vi "Teleop.vi"(10 "Match Info":T1={"Autonomous Elapsed Seconds"=0.0, "TeleOp Elapsed Seconds"=0.0, "Disabled Elapsed Seconds"=0.0, "Visited Autonomous"=FALSE, "Visited TeleOp"=FALSE, "Visited Disabled"=FALSE, "Autonomous Settings"={"Autonomous Style"=enum."Independent", "VI Refnum"=refnum}}, 11 "Call Context":T2) -> ()   [LabVIEW 2018]
doc: "This VI is called for each enabled TeleOp packet received from the DS. It is typically used to read from joysticks and other inputs and update I/O or setpoints for timed control loops. It should complete and return within 20 milliseconds or risk missing DS packets."
uses:
  <vilib>/Rock Robotics/WPI/DriverStation/WPI_DriverStationDerivedRobotMode.ctl
  <vilib>/Rock Robotics/WPI/DriverStation/WPI_DriverStationMatch Info.ctl
  <vilib>/Rock Robotics/WPI/Joystick/WPI_JoystickDeviceEnum.ctl
  <vilib>/addons/control/pid/pid.llb/PID (DBL).vi
  <vilib>/addons/control/pid/NI_PID_pid.lvlib
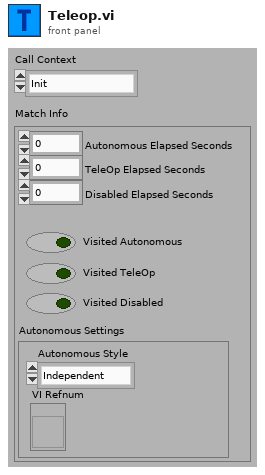
[diagram p1: front panel]
types:
  T1 = typedef "WPI_DriverStationMatch Info.ctl" = cluster{"Autonomous Elapsed Seconds":dbl, "TeleOp Elapsed Seconds":dbl, "Disabled Elapsed Seconds":dbl, "Visited Autonomous":bool, "Visited TeleOp":bool, "Visited Disabled":bool, "Autonomous Settings":cluster{"Autonomous Style":enum16{"Iterative", "Independent"}, "VI Refnum":refnum<vi>}}
  T2 = typedef "WPI_DriverStationDerivedRobotMode.ctl" = enum16{"Init", "Execute", "Stop"}
  T3 = typedef "WPI_JoystickDeviceEnum.ctl" = enum16{"USB 0", "USB 1", "USB 2", "USB 3", "USB 4", "USB 5"}
  T4 = cluster{"Autonomous Style":enum16{"Iterative", "Independent"}, "VI Refnum":refnum<vi>}
  T5 = typedef "Command Status Info.ctl" = cluster{"Name":string, "Status":T6, "notifier out":T7}
  T6 = typedef "Completion Status.ctl" = enum16{"Successful", "Aborted", "Incomplete"}
  T7 = typedef "Completion Notifier.ctl" = refnum<notifier>
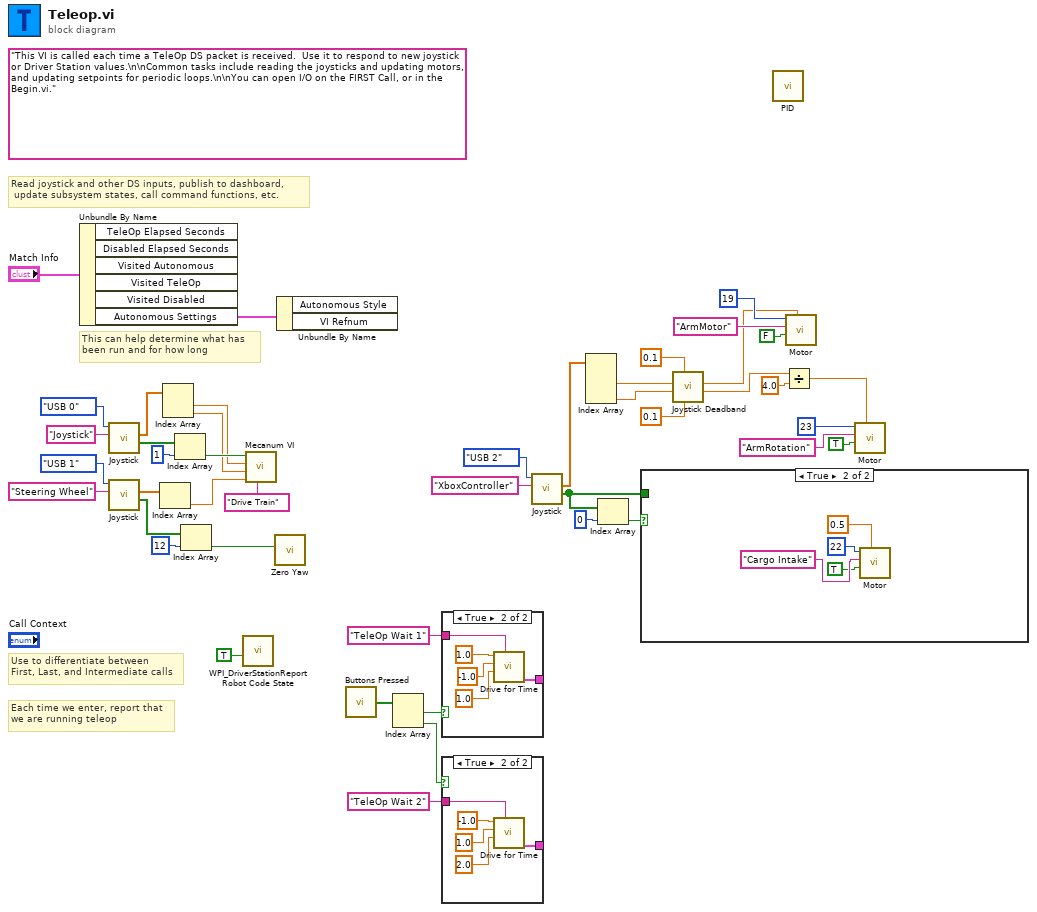
[diagram p0: block diagram]
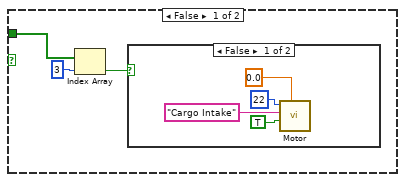
[diagram p2: hidden frame]
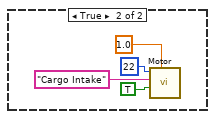
[diagram p3: hidden frame]
diagram:
  (unwired) "This VI is called each time a TeleOp DS packet is received.  Use it to respond to new joystick or Driver Station values.\n\nCommon tasks include reading the joysticks and updating motors, and updating setpoints for periodic loops.\n\nYou can open I/O on the FIRST Call, or in the Begin.vi."
  # "Read joystick and other DS inputs, publish to dashboard,\n update subsystem states, call command functions, etc."
  # "Each time we enter, report that\nwe are running teleop"
  # "Use to differentiate between\nFirst, Last, and Intermediate calls"
  # "This can help determine what has\nbeen run and for how long"
  n1 = Unbundle By Name("Match Info") -> ("Autonomous Settings"=w6:T4)  [unwired: 5 out]
  n2 = call "Joystick.vi"("Refnum Name"="Joystick", "JoystickDevice"=WPI_JoystickDeviceEnum."USB 0") -> ("Buttons"=w17:bool[], "Axes"=w35:dbl[])  [unwired: 7 in, 1 out]
  n3 = call "Joystick.vi"("Refnum Name"="Steering Wheel", "JoystickDevice"=WPI_JoystickDeviceEnum."USB 1") -> ("Buttons"=w19:bool[], "Axes"=w32:dbl[])  [unwired: 7 in, 1 out]
  n4 = Index Array(array=w32) -> (element=w2:dbl)  [unwired: 1 in]
  n5 = Index Array(array=w35) -> (element #1=w4:dbl, element #2=w3:dbl)  [unwired: 2 in]
  n6 = Index Array(array=w17, index=1) -> (element=w5:bool)
  n7 = Index Array(array=w19, index=12) -> (element=w15:bool)
  n8 = call <vilib>:"WPI_DriverStationReport Robot Code State.vi"("TeleOp"=TRUE ("Autonomous")) -> ()  [unwired: 10 in, 1 out]
  n9 = call "Mecanum VI.vi"("Drive Refnum"="Drive Train" ("refnum name"), "Z Value"=w2, "Y Value"=w3, "X Value"=w4, "Button Input"=w5) -> ()  [unwired: 7 in]
  n10 = call <vilib>:"Zero Yaw.vi"("Zero"=w15) -> ()  [unwired: 11 in]
  n11 = Unbundle By Name(w6) -> ()  [unwired: 2 out]
  n12 = call "Buttons Pressed.vi"() -> ("Button Presses"=w40:bool[])  [unwired: 1 in]
  n13 = Index Array(array=w40) -> (element #1=w39:bool, element #2=w38:bool)  [unwired: 2 in]
  n14 = case shown="True" w39 {
    tunnel: [_ w48] -> _
    tunnel: "TeleOp Wait 1" ("Description") -> [_ w47]
    frame False {
    }
    frame True {
      n15 = call "Drive for Time.vi"("Description"=w47, "Seconds"=1.0, "Right Speed"=-1.0, "Left Speed"=1.0) -> ("Command Info Out"=w48:T5)  [unwired: 7 in]
    }
  }
  n16 = case shown="True" w38 {
    tunnel: [_ w52] -> _
    tunnel: "TeleOp Wait 2" ("Description") -> [_ w51]
    frame False {
    }
    frame True {
      n17 = call "Drive for Time.vi"("Description"=w51, "Seconds"=2.0, "Right Speed"=1.0, "Left Speed"=-1.0) -> ("Command Info Out"=w52:T5)  [unwired: 7 in]
    }
  }
  n18 = call "Joystick.vi"("Refnum Name"="XboxController", "JoystickDevice"=WPI_JoystickDeviceEnum."USB 2") -> ("Buttons"=w20:bool[], "Axes"=w29:dbl[])  [unwired: 7 in, 1 out]
  n19 = Index Array(array=w29) -> (element #2=w25:dbl, element #4=w11:dbl)  [unwired: 4 in, 2 out]
  n20 = Index Array(array=w20, index=0) -> (element=w21:bool)
  n21 = case shown="True" w21 {
    tunnel: w20 -> [w56 _]
    frame False {
      n22 = Index Array(array=w56, index=3) -> (element=w55:bool)
      n23 = case shown="False" w55 {
        frame False {
          n24 = call "Motor.vi"("Motor Input"=0.0, "Victor SPX?"=TRUE, "Refnum Name"="Cargo Intake", "Device Number"=u8 22) -> ()  [unwired: 7 in, 1 out]
        }
        frame True {
          n25 = call "Motor.vi"("Motor Input"=1.0, "Victor SPX?"=TRUE, "Refnum Name"="Cargo Intake", "Device Number"=u8 22) -> ()  [unwired: 7 in, 1 out]
        }
      }
    }
    frame True {
      n26 = call "Motor.vi"("Motor Input"=0.5, "Victor SPX?"=TRUE, "Refnum Name"="Cargo Intake", "Device Number"=u8 22) -> ()  [unwired: 7 in, 1 out]
    }
  }
  n27 = call "Joystick Deadband.vi"("Z Deadband"=0.1, "X Y Deadband"=0.1, "Z"=w11, "Y"=w25) -> ("Z Out"=w9:dbl, "Y Out"=w24:dbl)  [unwired: 5 in, 1 out]
  n28 = call-poly <vilib>:"PID.vi"() -> ()  [unwired: 10 in, 2 out]
  n29 = Divide(x=w9, y=4.0) -> (x/y=w7:dbl)
  n30 = call "Motor.vi"("Motor Input"=w24, "Victor SPX?"=FALSE, "Refnum Name"="ArmMotor", "Device Number"=u8 19) -> ()  [unwired: 7 in, 1 out]
  n31 = call "Motor.vi"("Motor Input"=w7, "Victor SPX?"=TRUE, "Refnum Name"="ArmRotation", "Device Number"=u8 23) -> ()  [unwired: 7 in, 1 out]
